vi "UI 2 Data Handler.vi"(8 "error in (no error)":errorcluster, 10 "UI 2 Data":T1, 11 "Current Val Data Set":cluster{"Acq Data":T4, "Post-Analysis Data":T5}) -> (0 "error out":errorcluster)   [LabVIEW 2014]
uses:
  Top Level/Shared Controls/UI Ref Arrays.ctl
  Top Level/Shared Controls/Acq Data.ctl
  Top Level/Shared Controls/Post-Analysis Data.ctl
  Private Controls/UI  2 Data.ctl
  Testing UI 2.lvlib
  Top Level/Shared Controls/Calculated Data.ctl
  File IO/Public Controls/General APU Info.ctl
  File IO/File IO.lvlib
  Top Level/Shared Controls/APU Setup File.ctl
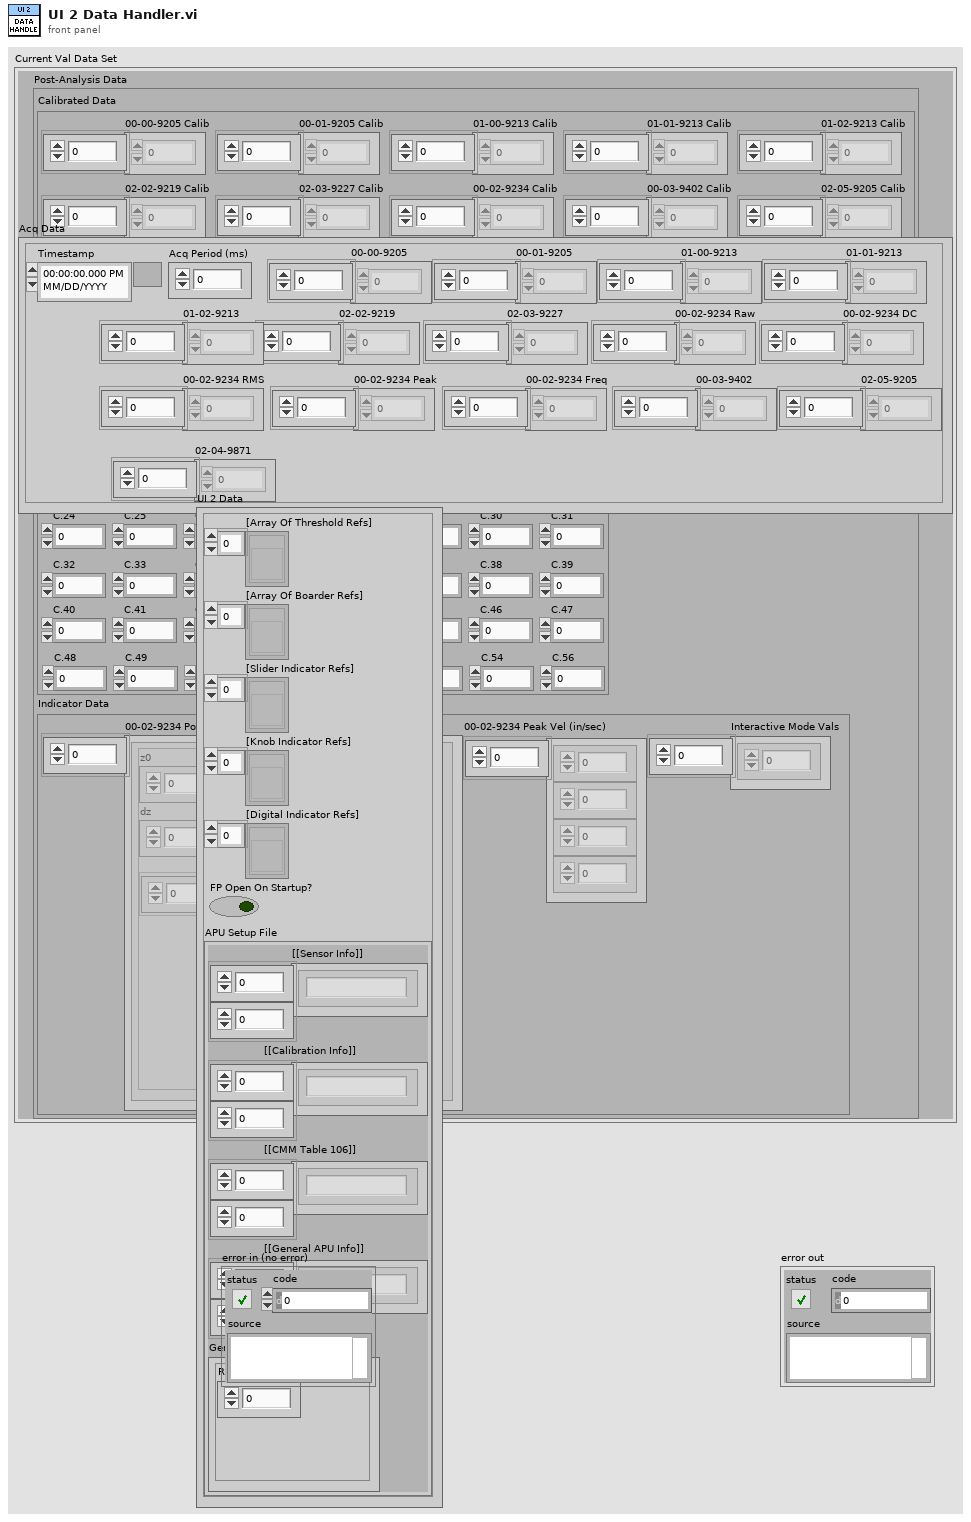
[diagram p1: front panel]
types:
  T1 = typedef "Testing UI 2.lvlib/UI  2 Data.ctl" = cluster{"[Array Of Threshold Refs]":refnum<vi>[], "[Array Of Boarder Refs]":refnum<vi>[], "[Slider Indicator Refs]":refnum<vi>[], "[Knob Indicator Refs]":refnum<vi>[], "[Digital Indicator Refs]":refnum<vi>[], "FP Open On Startup?":bool, "APU Setup File":T2}
  T2 = typedef "APU Setup File.ctl" = cluster{"[[Sensor Info]]":string[][], "[[Calibration Info]]":string[][], "[[CMM Table 106]]":string[][], "[[General APU Info]]":string[][], "General APU Information":T3}
  T3 = typedef "File IO.lvlib/General APU Info.ctl" = cluster{"Run Count":u64}
  T4 = typedef "Acq Data.ctl" = cluster{"Timestamp":timestamp, "Acq Period (ms)":i64, "00-00-9205":dbl[], "00-01-9205":dbl[], "01-00-9213":dbl[], "01-01-9213":dbl[], "01-02-9213":dbl[], "02-02-9219":dbl[], "02-03-9227":dbl[], "00-02-9234 Raw":dbl[], "00-02-9234 DC":dbl[], "00-02-9234 RMS":dbl[], "00-02-9234 Peak":dbl[], "00-02-9234 Freq":dbl[], "00-03-9402":dbl[], "02-05-9205":dbl[], "02-04-9871":dbl[]}
  T5 = typedef "Post-Analysis Data.ctl" = cluster{"Calibrated Data":cluster{"00-00-9205 Calib":dbl[], "00-01-9205 Calib":dbl[], "01-00-9213 Calib":dbl[], "01-01-9213 Calib":dbl[], "01-02-9213 Calib":dbl[], "02-02-9219 Calib":dbl[], "02-03-9227 Calib":dbl[], "00-02-9234 Calib":dbl[], "00-03-9402 Calib":dbl[], "02-05-9205 Calib":dbl[], "02-04-9871 2DArray":dbl[][]}, "Calculated Data":T6, "Indicator Data":cluster{"00-02-9234 Power Spectras":cluster{"z0":dbl, "dz":dbl, "waveforms":cluster{"f0":dbl, "df":dbl, "magnitude":dbl[]}[]}[], "00-02-9234 Peak Vel (in/sec)":dbl[], "Interactive Mode Vals":dbl[]}}
  T6 = typedef "Calculated Data.ctl" = cluster{"C.00":dbl, "C.01":dbl, "C.02":dbl, "C.03":dbl, "C.04":dbl, "C.05":dbl, "C.06":dbl, "C.07":dbl, "C.08":dbl, "C.09":dbl, "C.10":dbl, "C.11":dbl, "C.12":dbl, "C.13":dbl, "C.14":dbl, "C.15":dbl, "C.16":dbl, "C.17":dbl, "C.18":dbl, "C.19":dbl, "C.20":dbl, "C.21":dbl, "C.22":dbl, "C.23":dbl, "C.24":dbl, "C.25":dbl, "C.26":dbl, "C.27":dbl, "C.28":dbl, "C.29":dbl, "C.30":dbl, "C.31":dbl, "C.32":dbl, "C.33":dbl, "C.34":dbl, "C.35":dbl, "C.36":dbl, "C.37":dbl, "C.38":dbl, "C.39":dbl, "C.40":dbl, "C.41":dbl, "C.42":dbl, "C.43":dbl, "C.44":dbl, "C.45":dbl, "C.46":dbl, "C.47":dbl, "C.48":dbl, "C.49":dbl, "C.50":dbl, "C.51":dbl, "C.52":dbl, "C.53":dbl, "C.54":dbl, "C.56":dbl}
  T7 = typedef "UI Ref Arrays.ctl" = cluster{"[Slider Indicator Refs]":refnum<vi>[], "[Knob Indicator Refs]":refnum<vi>[], "[Digital Indicator Refs]":refnum<vi>[], "[[Sensor Info]]":string[][], "[Bool Indicator Refs]":refnum<vi>[]}
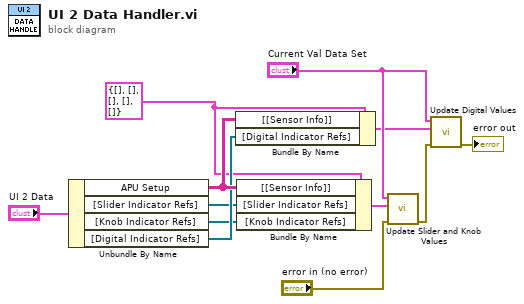
[diagram p0: block diagram]
diagram:
  w9 = T7 {"[Slider Indicator Refs]"=[], "[Knob Indicator Refs]"=[], "[Digital Indicator Refs]"=[], "[[Sensor Info]]"=[], "[Bool Indicator Refs]"=[]} ("Ref Data Array")
  n1 = Unbundle By Name("UI 2 Data") -> ("APU Setup"=w11:string[][], "[Slider Indicator Refs]"=w4:refnum<vi>[], "[Knob Indicator Refs]"=w5:refnum<vi>[], "[Digital Indicator Refs]"=w10:refnum<vi>[])
  n2 = Bundle By Name(cluster=w9, "[[Sensor Info]]"=w11, "[Digital Indicator Refs]"=w10) -> (w7:T7)
  n3 = Bundle By Name(cluster=w9, "[[Sensor Info]]"=w11, "[Slider Indicator Refs]"=w4, "[Knob Indicator Refs]"=w5) -> (w2:T7)
  n4 = call "Update Slider and Knob Values.vi"("error in"="error in (no error)", "Ref Data Array"=w2, "Current Val Data Set"="Current Val Data Set") -> ("error out"=w6:errorcluster)  [unwired: 6 in, 2 out]
  n5 = call "Update Digital Values.vi"("error in (no error)"=w6, "Ref Data Array"=w7, "Current Val Data Set"="Current Val Data Set") -> ("error out"=→"error out":errorcluster)  [unwired: 6 in, 2 out]
